vi "锁相采集.vi"(0 "VISA resource name":refnum<visa-resource-name> caption="VISA资源名称") -> (1 "输出":dbl, 2 "VISA资源名称输出":refnum<visa-resource-name>)   [LabVIEW 2016]
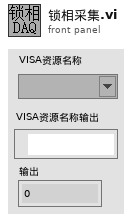
[diagram p1: front panel]
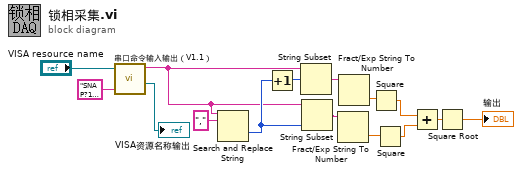
[diagram p0: block diagram]
diagram:
  n1 = call "串口命令输入输出（V1.1）.vi"("VISA resource name"="VISA resource name", "string to write"="SNAP?1,2\n") -> ("read string"=w3:string, "VISA资源名称输出"=→"VISA资源名称输出":refnum<visa-resource-name>)  [unwired: 1 in, 2 out]
  n2 = Search and Replace String(input string=w3, search string="," ("搜索字符串")) -> (offset past replacement=w12:i32)  [unwired: 6 in, 3 out]
  n3 = Increment(x=w12) -> (x+1=w13:i32)
  n4 = String Subset(string=w3, offset (0)=w13) -> (substring=w11:string)  [unwired: 1 in]
  n5 = String Subset(string=w3, length (rest)=w12) -> (substring=w10:string)  [unwired: 1 in]
  n6 = Fract/Exp String To Number(string=w10) -> (number=w8:dbl)  [unwired: 3 in, 1 out]
  n7 = Fract/Exp String To Number(string=w11) -> (number=w9:dbl)  [unwired: 3 in, 1 out]
  n8 = Square(x=w9) -> (x^2=w5:dbl)
  n9 = Square(x=w8) -> (x^2=w7:dbl)
  n10 = Add(x=w5, y=w7) -> (x+y=w6:dbl)
  n11 = Square Root(x=w6) -> (sqrt(x)=→"输出":dbl)
